vi "Stop Stream.vi"(8 "error in (no error)":errorcluster, 11 "TCS in":refnum<class "TCS.lvclass">) -> (0 "error out":errorcluster, 3 "TCS out":refnum<class "TCS.lvclass">)   [LabVIEW 2018, in "TCS.lvclass"]
uses:
  TCS.lvclass
  TCS.lvclass/TCS.ctl
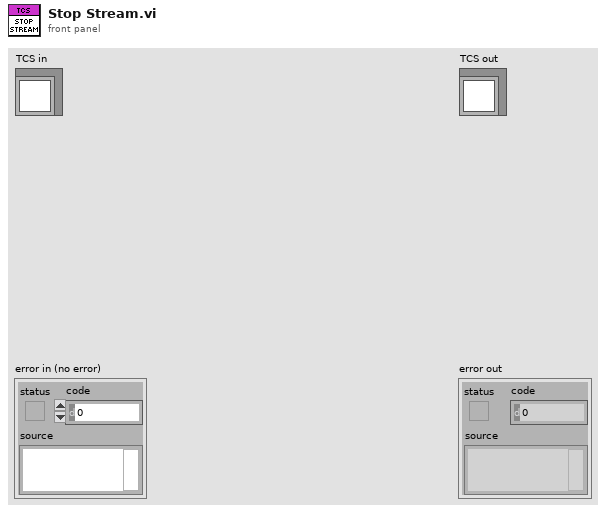
[diagram p1: front panel]
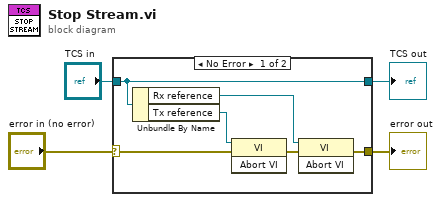
[diagram p0: block diagram]
diagram:
  n1 = case shown="No Error" "error in (no error)" {
    selector: "error in (no error)" -> [w6 w12]
    tunnel: [w5 w12] -> w3
    tunnel: [w7 w11] -> w1
    tunnel: "TCS in" -> [w7 w11]
    frame No Error {
      n2 = Unbundle By Name(w7) -> ("Rx reference"=w10:refnum<vi>, "Tx reference"=w9:refnum<vi>)
      n3 = invoke class="VI" method="Abort VI"(reference=w9, error in=w6) -> (error out=w8:errorcluster)  [unwired: 1 in, 2 out]
      n4 = invoke class="VI" method="Abort VI"(reference=w10, error in=w8) -> (error out=w5:errorcluster)  [unwired: 1 in, 2 out]
    }
    frame Error {
    }
  }
  "error out" <- w3
  "TCS out" <- w1
